vi "Acquire.vi"(8 "error in (no error)":errorcluster, 10 "Data Queue":refnum<queue>, 11 "Hardware Resources in":T1={"State"=enum."Idle S3DK", "Settings"="", "Status"={"Online"=FALSE, "Buffer"=FALSE, "Config"=FALSE, "Connect"=FALSE}, "S3DK"={"Signals"={"Phasor"=[], "Analog"=[], "Digital"=[]}}, "Tick"=0}) -> (0 "error out":errorcluster, 3 "Hardware Resources out":T1={"State"=enum."Idle S3DK", "Settings"="", "Status"={"Online"=FALSE, "Buffer"=FALSE, "Config"=FALSE, "Connect"=FALSE}, "S3DK"={"Signals"={"Phasor"=[], "Analog"=[], "Digital"=[]}}, "Tick"=0})   [LabVIEW 2017, in "Acquisition.lvlib"]
doc: "Perform the acquisition. Replace the contents of this diagram with calls to acquisition hardware."
uses:
  Acquisition.lvlib
  Acquisition Settings.ctl
  Acquisition State.ctl
  support/libs/PMU Buffer/Buffer DATA cluster.ctl
  support/libs/PMU Buffer/PMU data buffer.lvlib
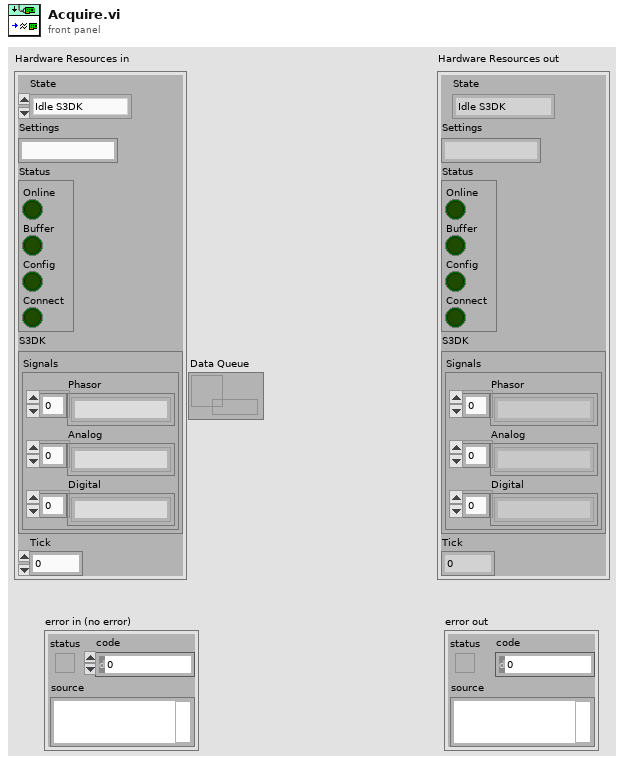
[diagram p1: front panel]
types:
  T1 = typedef "Acquisition.lvlib/Acquisition Settings.ctl" = cluster{"State":T2, "Settings":string, "Status":cluster{"Online":bool, "Buffer":bool, "Config":bool, "Connect":bool}, "S3DK":cluster{"Signals":cluster{"Phasor":string[], "Analog":string[], "Digital":string[]}}, "Tick":u32}
  T2 = typedef "Acquisition.lvlib/Acquisition State.ctl" = enum16{"Idle", "Idle S3DK", "Acquiring S3DK", "Idle CSV", "Acquiring CSV"}
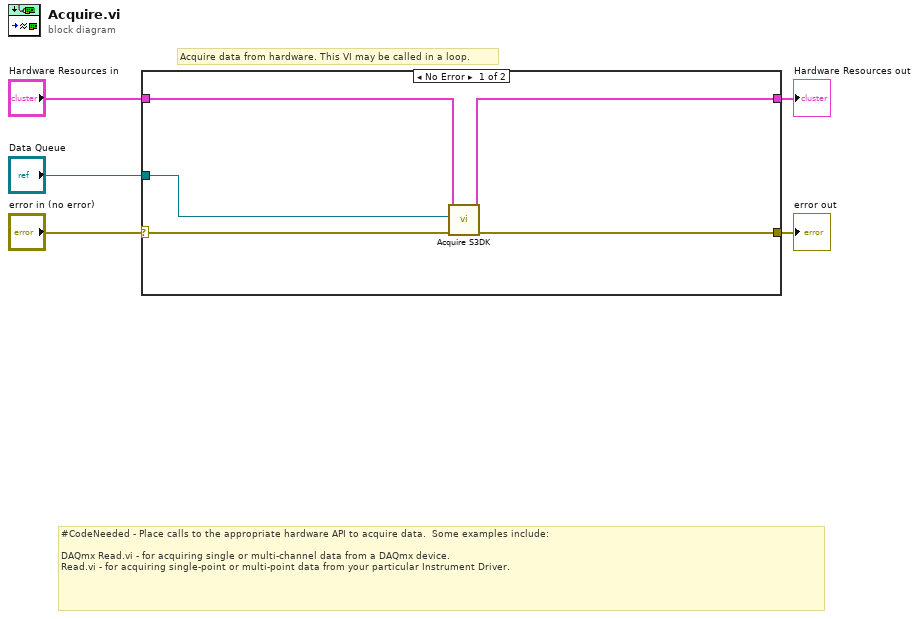
[diagram p0: block diagram]
diagram:
  # "Acquire data from hardware. This VI may be called in a loop."
  # "#CodeNeeded - Place calls to the appropriate hardware API to acquire data.  Some examples include:\n\nDAQmx Read.vi - for acquiring single or multi-channel data from a DAQmx device.\nRead.vi - for acquiring single-point or multi-point data from your particular Instrument Driver."
  n1 = case shown="No Error" "error in (no error)" {
    selector: "error in (no error)" -> [w10 w11]
    tunnel: [w9 w11] -> w4
    tunnel: "Hardware Resources in" -> [w7 w12]
    tunnel: [w6 w12] -> w2
    tunnel: "Data Queue" -> [w8 _]
    frame No Error {
      n2 = call "Acquire S3DK.vi"("error in (no error)"=w10, "DATA IN"=w8, "Hardware Resources in"=w7) -> ("error out"=w9:errorcluster, "Hardware Resources out"=w6:T1)  [unwired: 7 in]
    }
    frame Error {
    }
  }
  "Hardware Resources out" <- w2
  "error out" <- w4
